vi "Delete Message.vi"(8 "error in (no error)":errorcluster, 10 "Receipt Handle":string, 11 "SQS in":refnum<class "Queue.lvclass">) -> (0 "error out":errorcluster, 3 "SQS out":refnum<class "Queue.lvclass">)   [LabVIEW 2015, in "NI_AWS_SQS.lvlib" / "Queue.lvclass"]
doc: "Deletes the specified message from the specified queue. You specify the message by using the message's receipt handle and not the MessageId you receive when you send the message. Even if the message is locked by another reader due to the visibility timeout setting, it is still deleted from the queue. If you leave a message in the queue for longer than the queue's configured retention period, Amazon SQS automatically deletes the message.\n\nNote\nThe receipt handle is associated with a specific instance of receiving the message. If you receive a message more than once, the receipt handle you get each time you receive the message is different. If you don't provide the most recently received receipt handle for the message when you use the DeleteMessage action, the request succeeds, but the message might not be deleted.\nFor standard queues, it is possible to receive a message even after you delete it. This might happen on rare occasions if one of the servers storing a copy of the message is unavailable when you send the request to delete the message. The copy remains on the server and might be returned to you on a subsequent receive request. You should ensure that your application is idempotent, so that receiving a message more than once does not cause issues."
uses:
  Queue.lvclass
  Core/HTTP Request/Name Value Pair.ctl
  Core/HTTP Request/Request Options.ctl
  Queue.lvclass/Queue.ctl
  Read Account Number.vi
  Read Name.vi
  Core/HTTP Request/HTTP Request.lvclass
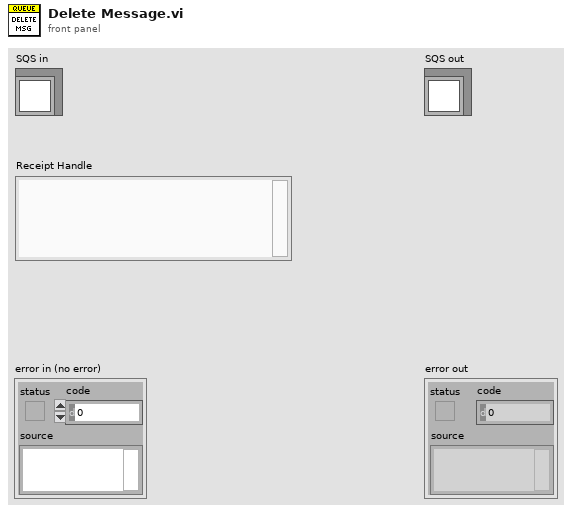
[diagram p1: front panel]
types:
  T1 = typedef "NI_AWS_Core.lvlib/HTTP Request.lvclass/Name Value Pair.ctl" = cluster{"name":string, "value":string}
  T2 = typedef "NI_AWS_Core.lvlib/HTTP Request.lvclass/Request Options.ctl" = cluster{"request headers":T1[], "request parameters":T1[], "request body":string}
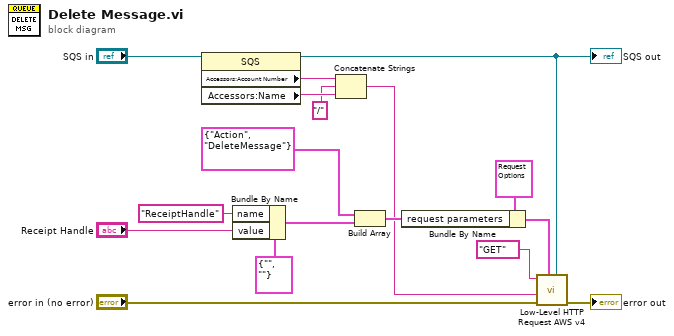
[diagram p0: block diagram]
diagram:
  n1 = property class="SQS"(reference="SQS in") -> (reference out=w10:refnum<class "Queue.lvclass">, "Accessors:Account Number"=w9:string, "Accessors:Name"=w8:string)  [unwired: 1 in, 1 out]
  "SQS out" <- w10
  n2 = Bundle By Name(cluster=T1 {"name"="", "value"=""} ("element"), "name"="ReceiptHandle", "value"="Receipt Handle") -> (w3:T1)
  n3 = Concatenate Strings(w9, "/", w8) -> (w6:string)
  n4 = Build Array(T1 {"name"="Action", "value"="DeleteMessage"} ("Cluster"), w3) -> (w11:T1[])
  n5 = Bundle By Name(cluster=T2 {"request headers"=[], "request parameters"=[{"name"="Action", "value"="ListQueues"}], "request body"=""} ("Request Options"), "request parameters"=w11) -> (w12:T2)
  n6 = call "Low-Level HTTP Request AWS v4.vi"("AWS Core"=w10, "Request Options"=w12, "error in (no error)"="error in (no error)", "URL Suffix"=w6, "HTTP-Verb"="GET") -> ("error out"=→"error out":errorcluster)  [unwired: 4 in, 2 out]
